vi "Derived Params Widget.vi"(8 "Error In":errorcluster) -> (0 "Error Out":errorcluster, 3 "New Derived Params Widget":refnum<class "Derived Params Widget.lvclass">)   [LabVIEW 2014, in "Derived Params Widget.lvclass"]
doc: "Constructs a new Derived Params Widget.\n\n\nCopyright (c) 2019 Sze Howe Koh.\nThis code is licensed under the MIT license."
uses:
  Derived Params Widget.lvclass
  <vilib>/addons/LQ/LQ Core/Qt/AlignmentFlag.ctl
  Derived Params Widget.lvclass/Derived Params Widget.ctl
  <vilib>/addons/LQ/Qt Widgets/QFormLayout/setLabelAlignment.vi
  <vilib>/addons/LQ/Qt Widgets/QAbstractSpinBox/setReadOnly.vi
  <vilib>/addons/LQ/Qt Widgets/QDoubleSpinBox/setSuffix.vi
  <vilib>/addons/LQ/Qt Widgets/QDoubleSpinBox/setMaximum.vi
  <vilib>/addons/LQ/Qt Widgets/QDoubleSpinBox/setMinimum.vi
  <vilib>/addons/LQ/Qt Widgets/QLabel/QLabel.lvclass
  <vilib>/addons/LQ/Qt Widgets/QFormLayout/QFormLayout.lvclass
  <vilib>/addons/LQ/Qt Widgets/QWidget/QWidget.lvclass
  <vilib>/addons/LQ/LQ Core/Qt/Qt.lvlib
  <vilib>/addons/LQ/Qt Widgets/QGroupBox/QGroupBox.lvclass
  <vilib>/addons/LQ/Qt Widgets/QDoubleSpinBox/QDoubleSpinBox.lvclass
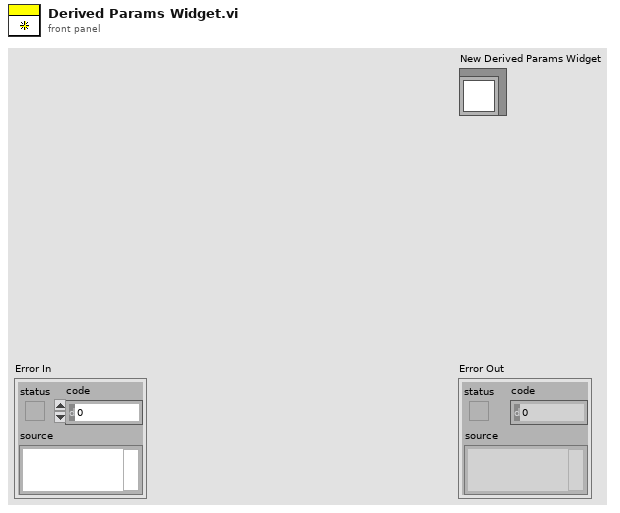
[diagram p1: front panel]
types:
  T1 = typedef "Qt.lvlib/AlignmentFlag.ctl" = i32
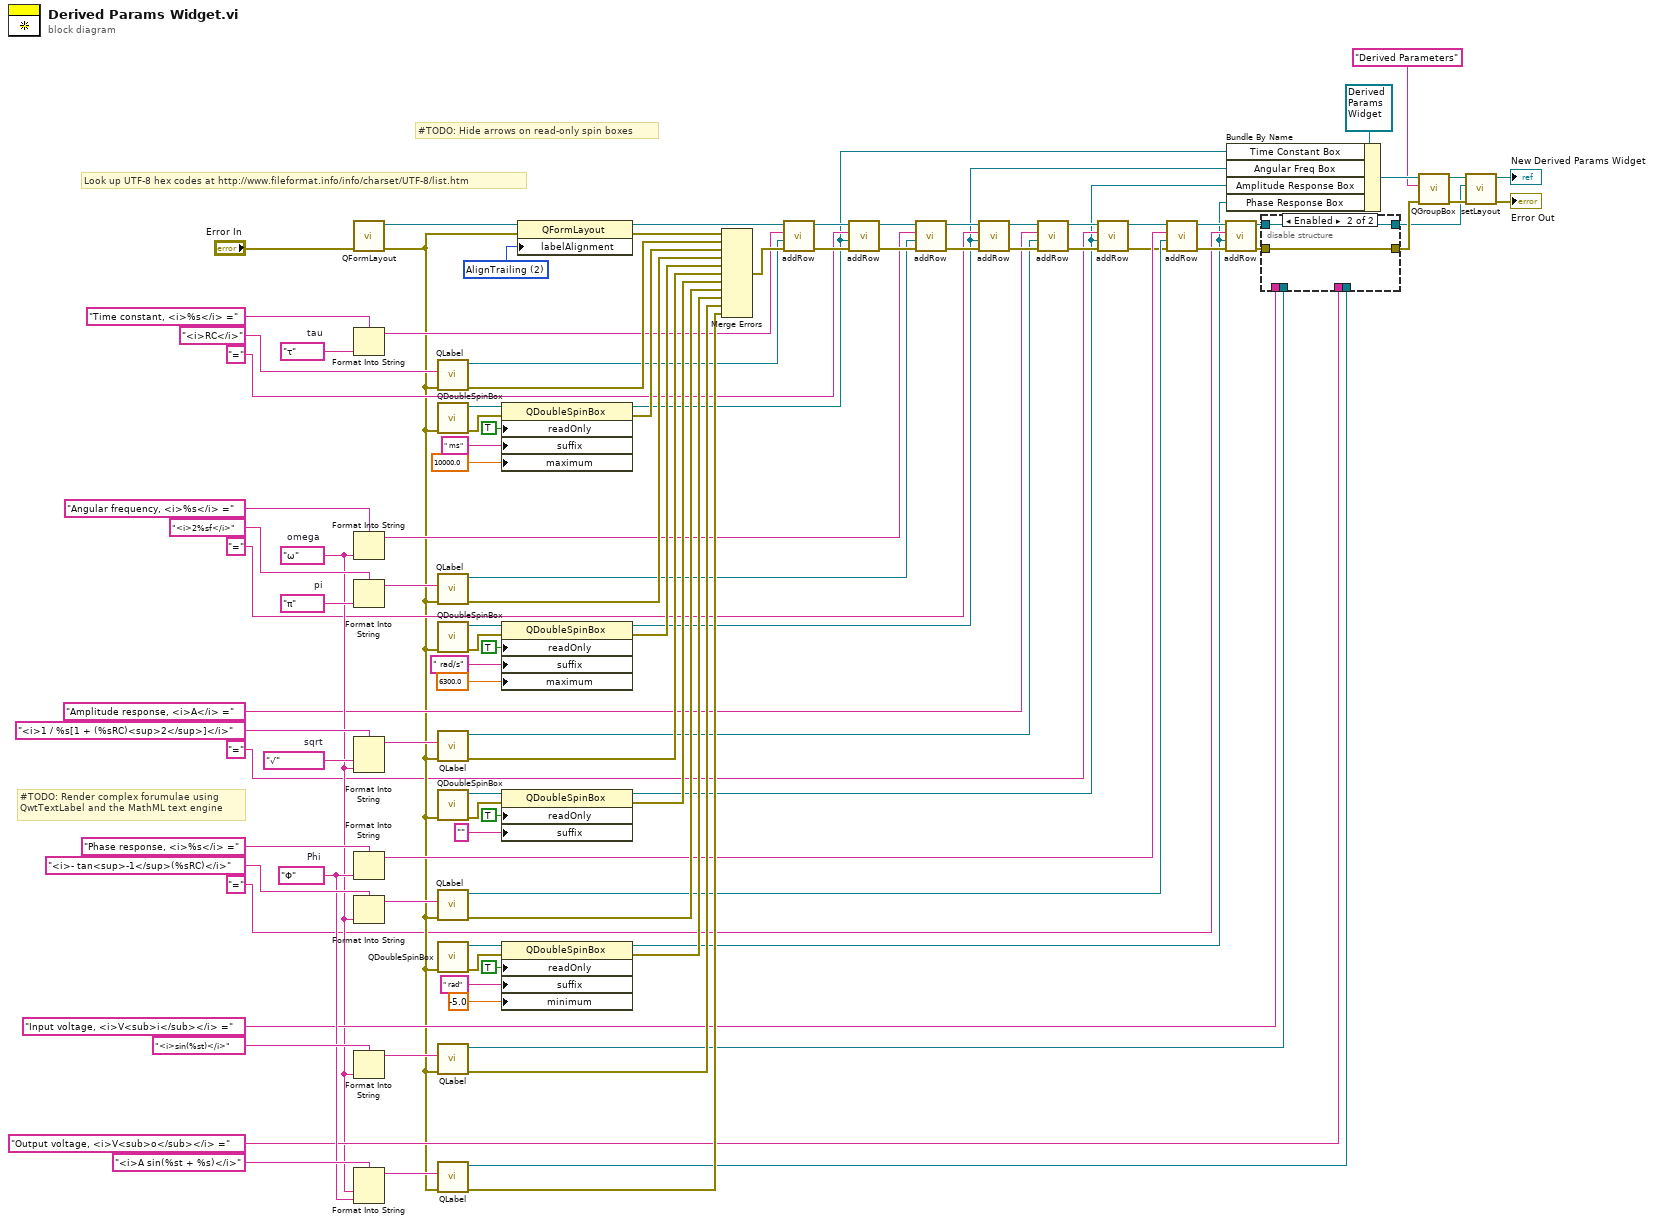
[diagram p0: block diagram]
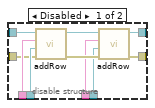
[diagram p2: hidden frame]
diagram:
  w44 = T1 2 items=["AlignLeading"=1, "AlignTrailing"=2, "AlignHCenter"=4, "AlignJustify"=8, "AlignAbsolute"=16, "AlignHorizontal_Mask"=31, "AlignTop"=32, "AlignBottom"=64, "AlignVCenter"=128, "AlignBaseline"=256, "AlignVertical_Mask"=480, "AlignCenter"=132] ("labelAlignment")
  w61 = "π"  # pi
  w74 = "τ"  # tau
  w81 = "√"  # sqrt
  w53 = "Φ"  # Phi
  w45 = "ω"  # omega
  # "#TODO: Hide arrows on read-only spin boxes"
  # "#TODO: Render complex forumulae using\nQwtTextLabel and the MathML text engine"
  # "Look up UTF-8 hex codes at http://www.fileformat.info/info/charset/UTF-8/list.htm"
  n1 = call <vilib>:"QFormLayout.vi"("Error In"="Error In") -> ("Error Out"=w24:errorcluster, "New QFormLayout"=w67:refnum<class "QFormLayout.lvclass">)  [unwired: 9 in]
  n2 = Format Into String(format string="Time constant, <i>%s</i> =" ("text"), w74) -> (resulting string=w72:string)  [unwired: 2 in, 1 out]
  n3 = Format Into String(format string="Angular frequency, <i>%s</i> =" ("text"), w45) -> (resulting string=w57:string)  [unwired: 2 in, 1 out]
  n4 = Format Into String(format string="<i>2%sf</i>" ("text"), w61) -> (resulting string=w59:string)  [unwired: 2 in, 1 out]
  n5 = Format Into String(format string="<i>1 / %s[1 + (%sRC)<sup>2</sup>]</i>" ("text"), w81, w45) -> (resulting string=w78:string)  [unwired: 2 in, 1 out]
  n6 = Format Into String(format string="Phase response, <i>%s</i> =" ("text"), w53) -> (resulting string=w52:string)  [unwired: 2 in, 1 out]
  n7 = Format Into String(format string="<i>- tan<sup>-1</sup>(%sRC)</i>" ("text"), w45) -> (resulting string=w77:string)  [unwired: 2 in, 1 out]
  n8 = Format Into String(format string="<i>sin(%st)</i>" ("text"), w45) -> (resulting string=w80:string)  [unwired: 2 in, 1 out]
  n9 = Format Into String(format string="<i>A sin(%st + %s)</i>" ("text"), w45, w53) -> (resulting string=w79:string)  [unwired: 2 in, 1 out]
  n10 = call <vilib>:"QLabel.vi"("Error In"=w24, "text"="<i>RC</i>") -> ("Error Out"=w90:errorcluster, "New QLabel"=w68:refnum<class "QLabel.lvclass">)  [unwired: 8 in]
  n11 = call <vilib>:"QDoubleSpinBox.vi"("Error In"=w24) -> ("Error Out"=w71:errorcluster, "New QDoubleSpinBox"=w29:refnum<class "QDoubleSpinBox.lvclass">)  [unwired: 9 in]
  n12 = call <vilib>:"QLabel.vi"("Error In"=w24, "text"=w59) -> ("Error Out"=w92:errorcluster, "New QLabel"=w58:refnum<class "QLabel.lvclass">)  [unwired: 8 in]
  n13 = call <vilib>:"QDoubleSpinBox.vi"("Error In"=w24) -> ("Error Out"=w60:errorcluster, "New QDoubleSpinBox"=w30:refnum<class "QDoubleSpinBox.lvclass">)  [unwired: 9 in]
  n14 = call <vilib>:"QLabel.vi"("Error In"=w24, "text"=w78) -> ("Error Out"=w88:errorcluster, "New QLabel"=w55:refnum<class "QLabel.lvclass">)  [unwired: 8 in]
  n15 = call <vilib>:"QDoubleSpinBox.vi"("Error In"=w24) -> ("Error Out"=w27:errorcluster, "New QDoubleSpinBox"=w28:refnum<class "QDoubleSpinBox.lvclass">)  [unwired: 9 in]
  n16 = call <vilib>:"QLabel.vi"("Error In"=w24, "text"=w77) -> ("Error Out"=w87:errorcluster, "New QLabel"=w51:refnum<class "QLabel.lvclass">)  [unwired: 8 in]
  n17 = call <vilib>:"QDoubleSpinBox.vi"("Error In"=w24) -> ("Error Out"=w25:errorcluster, "New QDoubleSpinBox"=w26:refnum<class "QDoubleSpinBox.lvclass">)  [unwired: 9 in]
  n18 = call <vilib>:"QLabel.vi"("Error In"=w24, "text"=w80) -> ("Error Out"=w86:errorcluster, "New QLabel"=w48:refnum<class "QLabel.lvclass">)  [unwired: 8 in]
  n19 = call <vilib>:"QLabel.vi"("Error In"=w24, "text"=w79) -> ("Error Out"=w85:errorcluster, "New QLabel"=w46:refnum<class "QLabel.lvclass">)  [unwired: 8 in]
  n20 = property class="QDoubleSpinBox"(reference=w29, error in=w71, "readOnly"=TRUE, "suffix"=" ms", "maximum"=10000.0) -> (reference out=w37:refnum<class "QDoubleSpinBox.lvclass">, error out=w89:errorcluster)
  n21 = property class="QDoubleSpinBox"(reference=w30, error in=w60, "readOnly"=TRUE, "suffix"=" rad/s", "maximum"=6300.0) -> (reference out=w36:refnum<class "QDoubleSpinBox.lvclass">, error out=w91:errorcluster)
  n22 = property class="QDoubleSpinBox"(reference=w28, error in=w27, "readOnly"=TRUE, "suffix"="") -> (reference out=w13:refnum<class "QDoubleSpinBox.lvclass">, error out=w100:errorcluster)
  n23 = property class="QDoubleSpinBox"(reference=w26, error in=w25, "readOnly"=TRUE, "suffix"=" rad", "minimum"=-5.0) -> (reference out=w12:refnum<class "QDoubleSpinBox.lvclass">, error out=w99:errorcluster)
  n24 = property class="QFormLayout"(reference=w67, error in=w24, "labelAlignment"=w44) -> (reference out=w66:refnum<class "QFormLayout.lvclass">, error out=w41:errorcluster)
  n25 = Merge Errors(w41, w90, w89, w92, w91, w88, w100, w87, w99, w86, w85) -> (w84:errorcluster)
  n26 = call <vilib>:"addRow.vi"("Error In"=w84, "field"=w68, "labelText"=w72, "QFormLayout In"=w66) -> ("Error Out"=w96:errorcluster, "QFormLayout Out"=w70:refnum<class "QFormLayout.lvclass">)  [unwired: 6 in]
  n27 = call <vilib>:"addRow.vi"("Error In"=w96, "field"=w37, "labelText"="=" ("suffix"), "QFormLayout In"=w70) -> ("Error Out"=w95:errorcluster, "QFormLayout Out"=w64:refnum<class "QFormLayout.lvclass">)  [unwired: 6 in]
  n28 = call <vilib>:"addRow.vi"("Error In"=w95, "field"=w58, "labelText"=w57, "QFormLayout In"=w64) -> ("Error Out"=w94:errorcluster, "QFormLayout Out"=w65:refnum<class "QFormLayout.lvclass">)  [unwired: 6 in]
  n29 = call <vilib>:"addRow.vi"("Error In"=w94, "field"=w36, "labelText"="=" ("suffix"), "QFormLayout In"=w65) -> ("Error Out"=w93:errorcluster, "QFormLayout Out"=w56:refnum<class "QFormLayout.lvclass">)  [unwired: 6 in]
  n30 = call <vilib>:"addRow.vi"("Error In"=w93, "field"=w55, "labelText"="Amplitude response, <i>A</i> =" ("text"), "QFormLayout In"=w56) -> ("Error Out"=w23:errorcluster, "QFormLayout Out"=w21:refnum<class "QFormLayout.lvclass">)  [unwired: 6 in]
  n31 = call <vilib>:"addRow.vi"("Error In"=w23, "field"=w13, "labelText"="=" ("suffix"), "QFormLayout In"=w21) -> ("Error Out"=w22:errorcluster, "QFormLayout Out"=w20:refnum<class "QFormLayout.lvclass">)  [unwired: 6 in]
  n32 = call <vilib>:"addRow.vi"("Error In"=w22, "field"=w51, "labelText"=w52, "QFormLayout In"=w20) -> ("Error Out"=w19:errorcluster, "QFormLayout Out"=w17:refnum<class "QFormLayout.lvclass">)  [unwired: 6 in]
  n33 = call <vilib>:"addRow.vi"("Error In"=w19, "field"=w12, "labelText"="=" ("suffix"), "QFormLayout In"=w17) -> ("Error Out"=w18:errorcluster, "QFormLayout Out"=w16:refnum<class "QFormLayout.lvclass">)  [unwired: 6 in]
  n34 = Bundle By Name(cluster=refnum<class "Derived Params Widget.lvclass"> refnum ("Derived Params Widget"), "Time Constant Box"=w37, "Angular Freq Box"=w36, "Amplitude Response Box"=w13, "Phase Response Box"=w12) -> (w35:refnum<class "Derived Params Widget.lvclass">)
  n35 = disable-structure shown="Enabled" {
    disable-tunnel: [w110 w111] -> w98
    disable-tunnel: [w107 w112] -> w50
    disable-tunnel: "Input voltage, <i>V<sub>i</sub></i> =" ("text") -> [w106 _]
    disable-tunnel: w48 -> [w105 _]
    disable-tunnel: "Output voltage, <i>V<sub>o</sub></i> =" ("text") -> [w104 _]
    disable-tunnel: w46 -> [w103 _]
    disable-tunnel: w18 -> [w102 w111]
    disable-tunnel: w16 -> [w101 w112]
    frame Disabled {
      n36 = call <vilib>:"addRow.vi"("Error In"=w102, "field"=w105, "labelText"=w106, "QFormLayout In"=w101) -> ("Error Out"=w109:errorcluster, "QFormLayout Out"=w108:refnum<class "QFormLayout.lvclass">)  [unwired: 6 in]
      n37 = call <vilib>:"addRow.vi"("Error In"=w109, "field"=w103, "labelText"=w104, "QFormLayout In"=w108) -> ("Error Out"=w110:errorcluster, "QFormLayout Out"=w107:refnum<class "QFormLayout.lvclass">)  [unwired: 6 in]
    }
    frame Enabled {
    }
  }
  n38 = call <vilib>:"QGroupBox.vi"("Error In"=w98, "title"="Derived Parameters", "Post-Bundled Subclass"=w35) -> ("Error Out"=w97:errorcluster, "New QGroupBox"=w34:refnum<class "Derived Params Widget.lvclass">)  [unwired: 7 in]
  n39 = call <vilib>:"setLayout.vi"("Error In"=w97, "layout"=w50, "QWidget In"=w34) -> ("Error Out"=→"Error Out":errorcluster, "QWidget Out"=→"New Derived Params Widget":refnum<class "Derived Params Widget.lvclass">)  [unwired: 7 in]
